vi "MB_TCP_7018_po.vi"(6 "N":i32, 9 "timeouts":T1={"conn_timeout"=1000, "reconn_timeout"=3000, "N attempt max"=3, "t_reset_TTL"=120000, "write_timeout"=10, "read_timeout"=500, "period"=100} {"t_reset_TTL" min=10 max=240000 step=1; "period" min=10 max=100000 step=1; "read_timeout" min=10 max=60000 step=1; "write_timeout" min=1 max=60000 step=1; "N attempt max" min=1 max=5 step=1; "reconn_timeout" min=10 max=240000 step=1; "conn_timeout" min=10 max=240000}, 10 "write enable":bool=TRUE, 11 "stop":bool) -> (0 "error out":errorcluster, 2 "errors":u32, 3 "Z3":u32)   [LabVIEW 2019]
uses:
  NI_modbus_upd/NI_modbus_upd.lvlib
  NI_modbus_upd.llb/MB Modbus Command.ctl
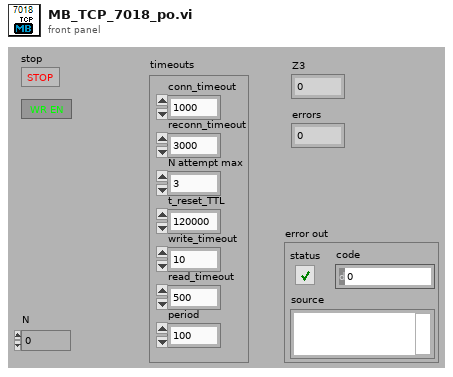
[diagram p1: front panel]
types:
  T1 = cluster{"conn_timeout":i32, "reconn_timeout":u32, "N attempt max":i32, "t_reset_TTL":u32, "write_timeout":i32, "read_timeout":i32, "period":u32}
  T2 = enum16{"Init", "Read", "Write", "Read inputs", "Read outputs"}
  T3 = enum16{"DI", "DO to write", "DO", "AI", "AO to write", "AO", "DI AI", "DI AO", "DO AI", "DO AO"}
  T4 = enum16{"Start", "Connect", "Write enable", "IP address", "Errors"}
  T5 = cluster{"Transaction ID":u16, "Protocol ID":u16, "Length":u16, "Unit ID":u8}
  T6 = typedef "MB Modbus Command.ctl" = cluster{"Function Code":u8, "Starting Address":u16, "Quantity":u16, "Data":u16[], "Discrete":bool[]}
  T7 = cluster{"Remote IP Address":string, "Remote Port":u16}
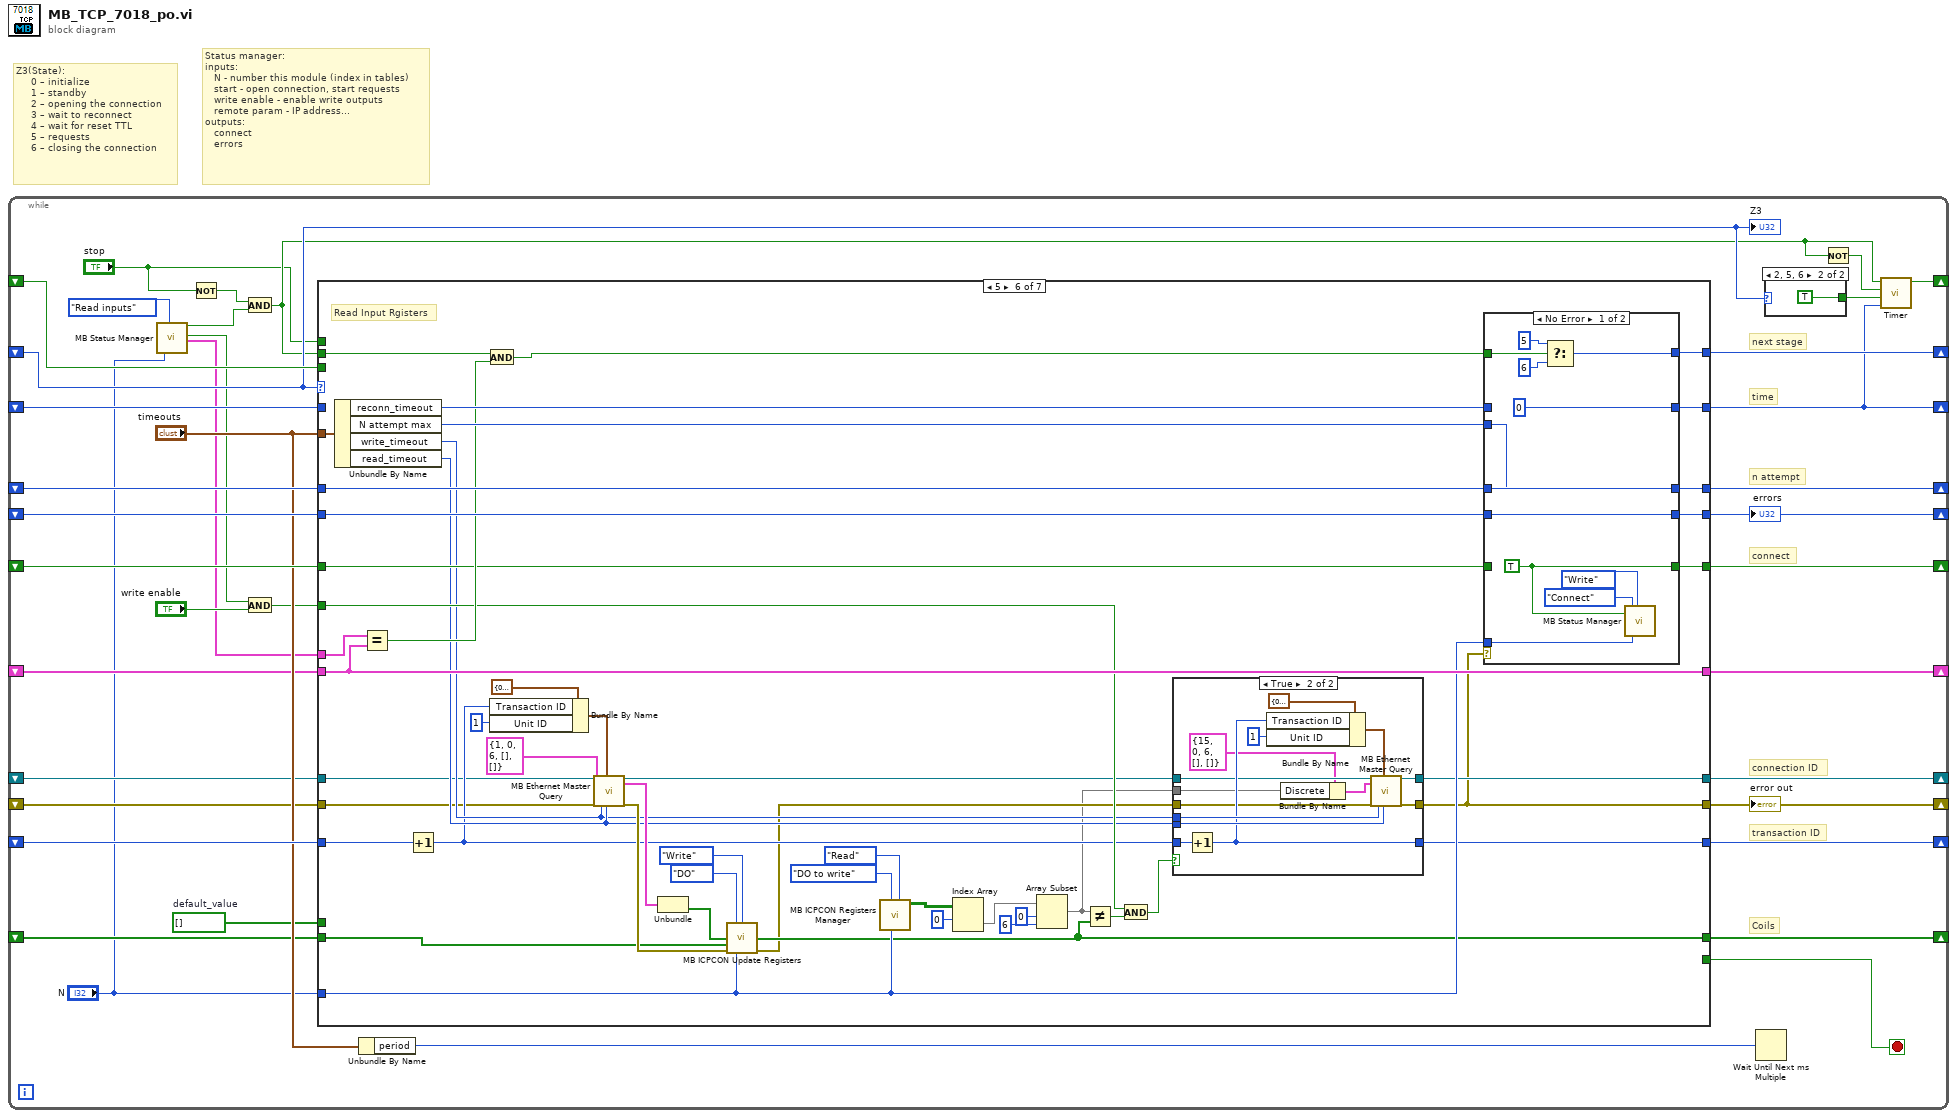
[diagram p0: block diagram]
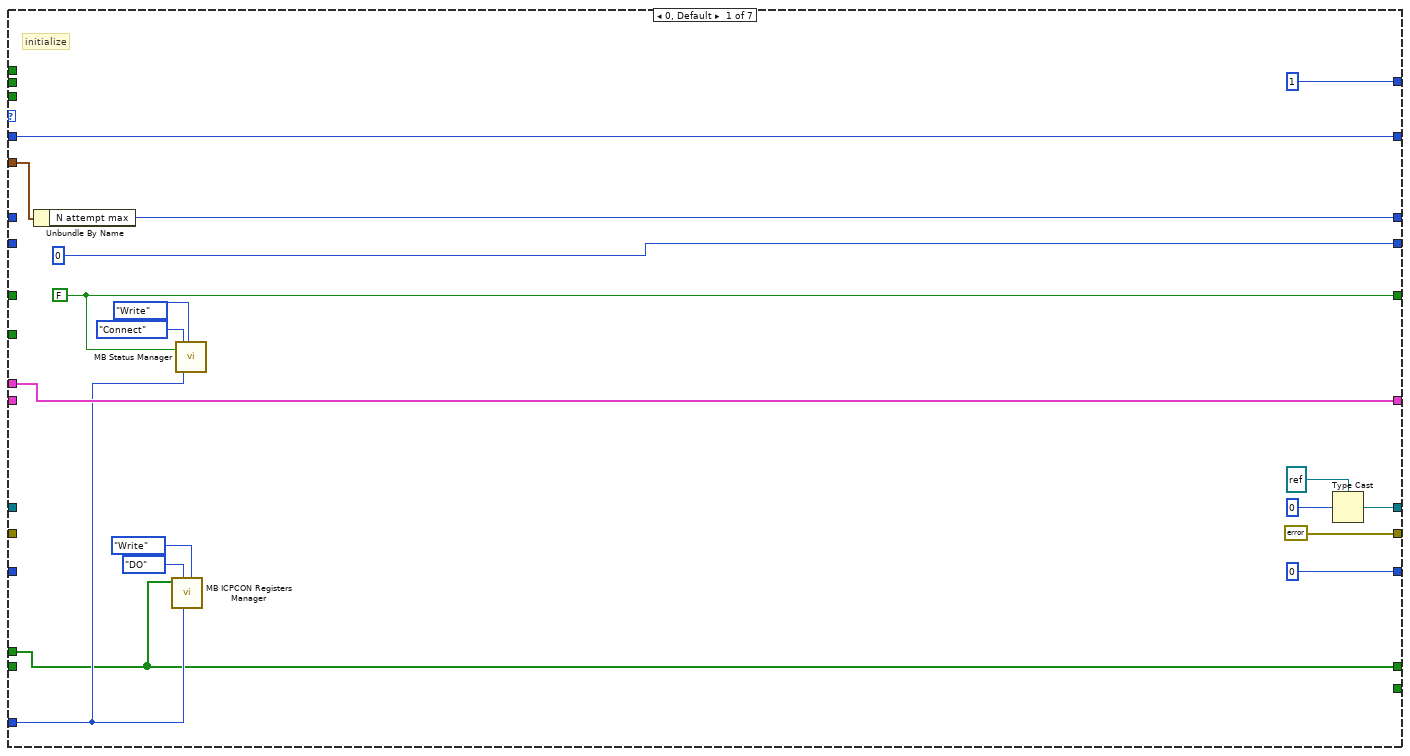
[diagram p2: hidden frame]
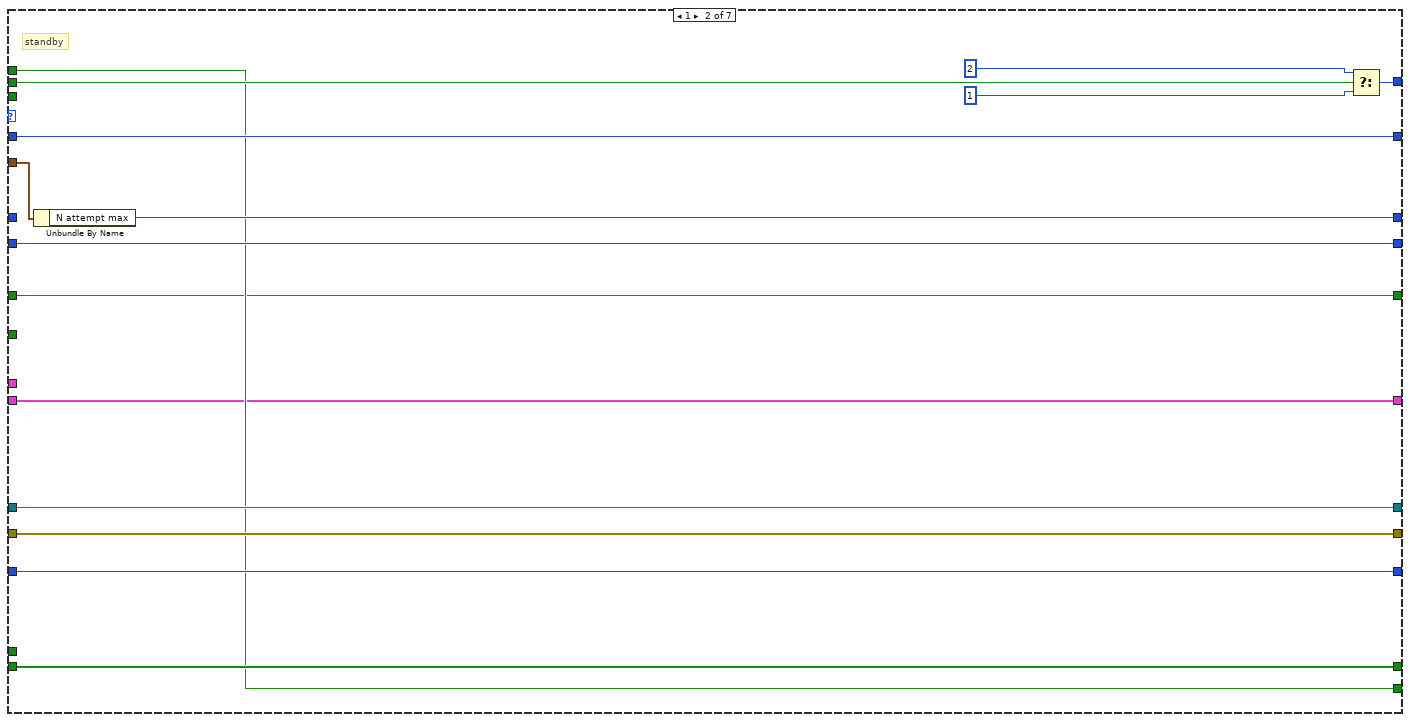
[diagram p3: hidden frame]
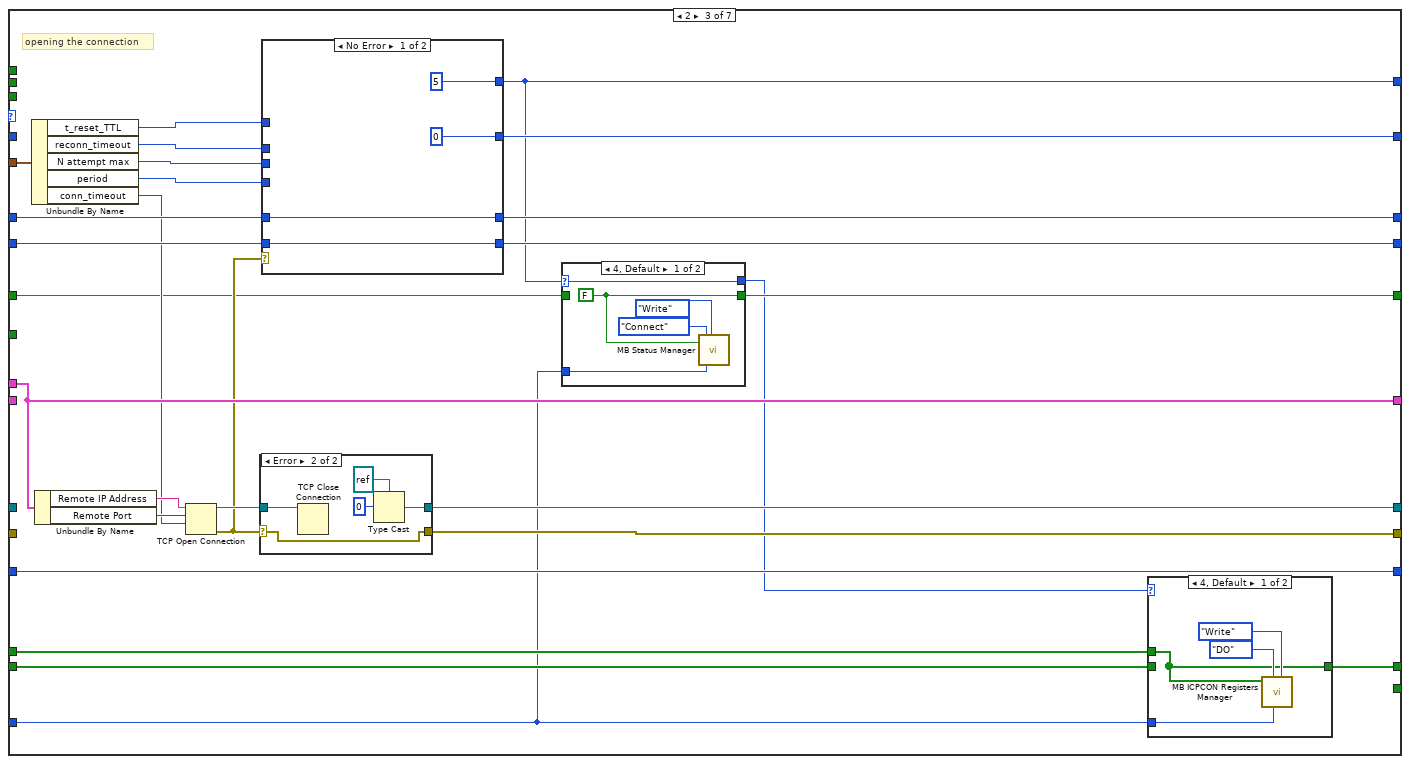
[diagram p4: hidden frame]
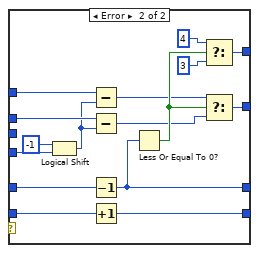
[diagram p7: hidden frame]
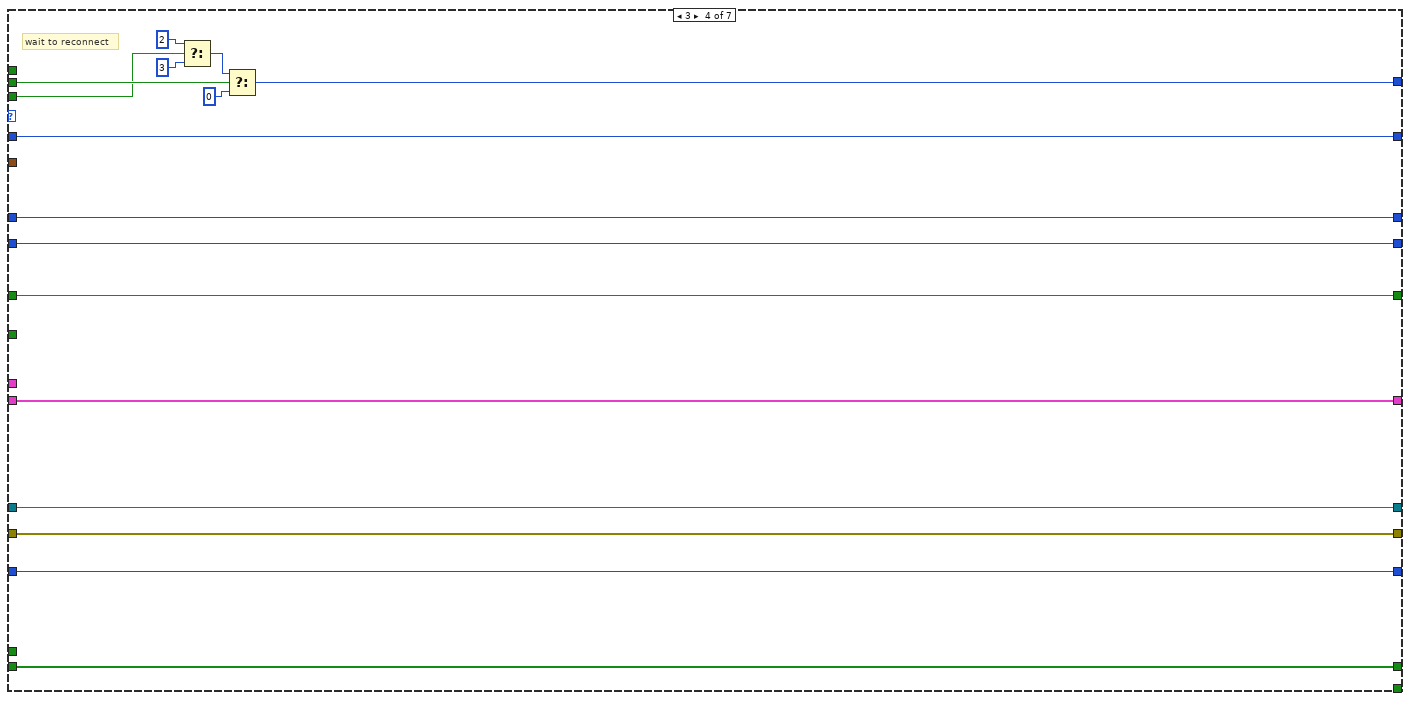
[diagram p9: hidden frame]
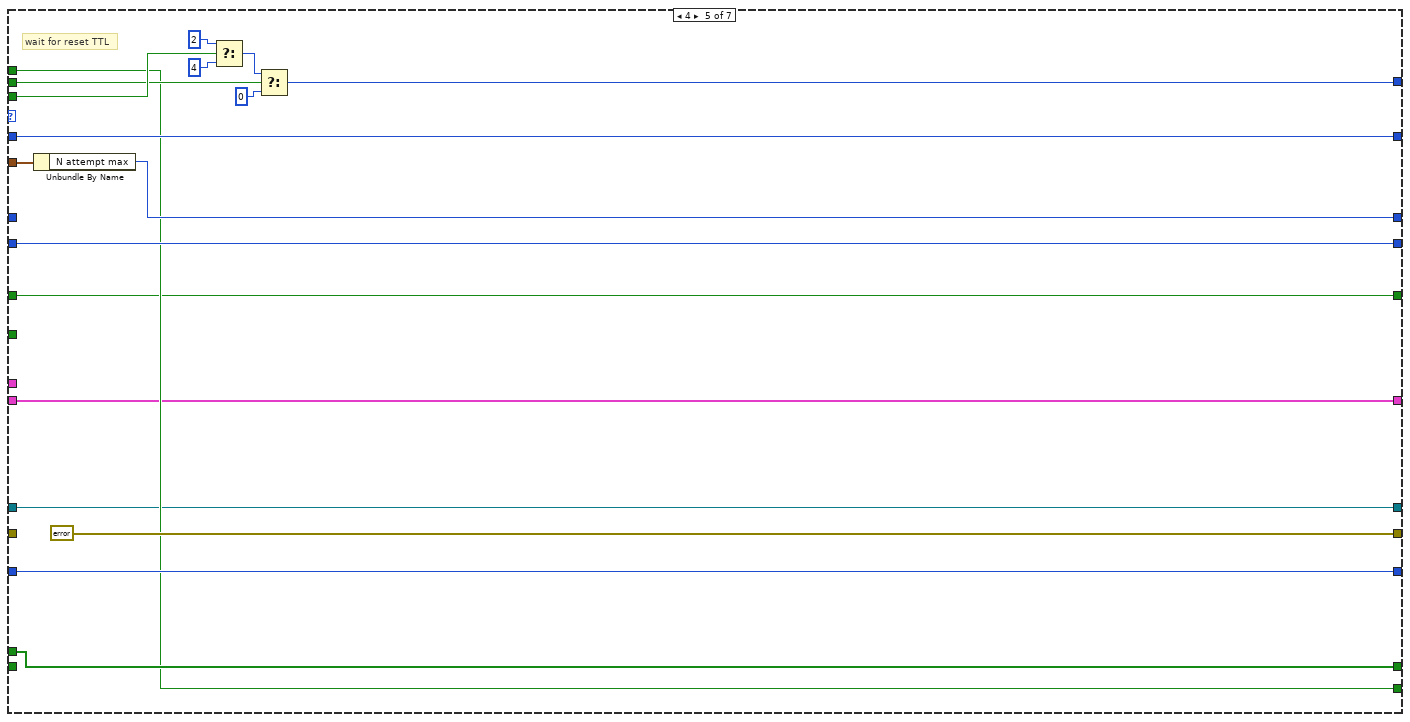
[diagram p10: hidden frame]
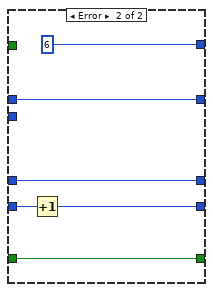
[diagram p12: hidden frame]
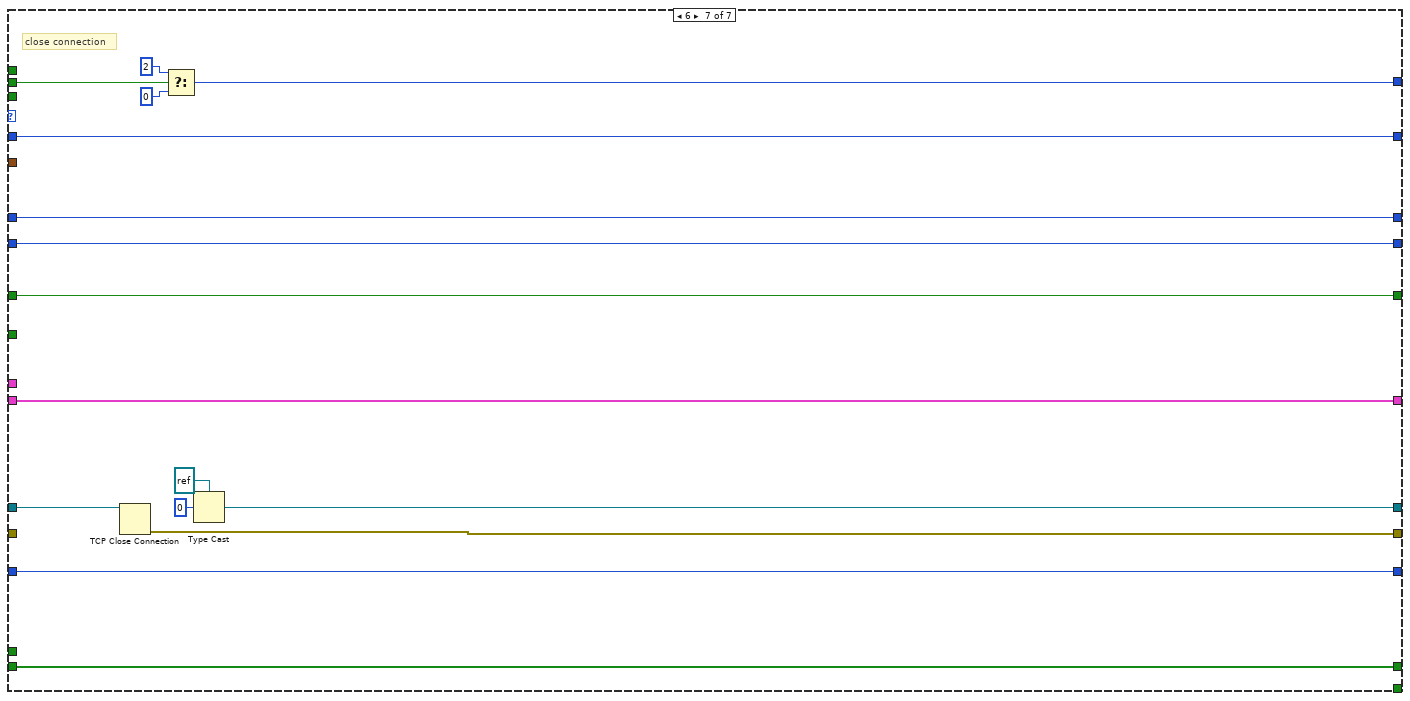
[diagram p13: hidden frame]
diagram:
  # "Status manager:\ninputs:\n   N - number this module (index in tables)\n   start - open connection, start requests\n   write enable - enable write outputs\n   remote param - IP address...\noutputs:\n   connect\n   errors"
  # "Z3(State):\n     0 – initialize \n     1 – standby\n     2 – opening the connection\n     3 – wait to reconnect\n     4 – wait for reset TTL\n     5 – requests\n     6 – closing the connection"
  n1 = while {
    shift-right: [w18] -> _
    shift-left: _ -> [w14]
    shift-right: [w17] -> _
    shift-left: _ -> [w37]
    shift-right: [w36] -> _
    shift-left: _ -> [w34]
    shift-right: [w35] -> _
    shift-left: _ -> [w33]
    shift-right: [w32] -> _
    shift-left: _ -> [w31]
    shift-right: [w30] -> _
    shift-left: _ -> [w19]
    shift-right: [w29] -> _
    shift-left: _ -> [w20]
    shift-right: [w28] -> _
    shift-left: _ -> [w27]
    shift-right: [w22] -> _
    shift-left: _ -> [w21]
    shift-right: [w16] -> _
    shift-left: _ -> [w15]
    shift-right: [w7] -> _
    shift-left: _ -> [w6]
    stop <- w10 stop-if-true
    w23 = bool[] []  # default_value
    # "Coils"
    # "connect"
    # "connection ID"
    # "transaction ID"
    # "n attempt"
    # "time"
    # "next stage"
    n2 = call "MB Status Manager.vi"("N"="N", "Function"=T2."Read inputs") -> ("start"=w4:bool, "write enable"=w3:bool, "Remote Param"=w2:T7)  [unwired: 12 in, 3 out]
    n3 = Not(x="stop") -> (.not. x?=w12:bool)
    n4 = And(x=w12, y=w4) -> (x .and. y?=w13:bool)
    n5 = And(x=w3, y="write enable") -> (x .and. y?=w9:bool)
    n6 = case shown="5" w14 {
      tunnel: [w54 w63 w79 w151 w156 w181 w268] -> w30
      tunnel: [errorcluster {"status"=FALSE, "code"=0, "source"=""} ("error out") w62 w77 w150 errorcluster {"status"=FALSE, "code"=0, "source"=""} ("error out") w180 w269] -> w29
      tunnel: w19 -> [_ w63 _ w151 w156 w173 w265]
      tunnel: w20 -> [_ w62 _ w150 _ w174 _]
      tunnel: [w42 w58 w75 w139 w155 w206 w256] -> w32
      tunnel: w31 -> [_ w58 w76 w139 w155 w207 w256]
      tunnel: w2 -> [w46 _ w82 _ _ w212 _]
      tunnel: w27 -> [_ w71 w98 w153 w171 w172 w270]
      tunnel: [u16 0 ("x") w71 w98 w153 w171 w183 w270] -> w28
      tunnel: [w48 w67 w93 w152 w167 w219 w262] -> w36
      tunnel: w34 -> [_ _ w94 w152 _ w219 w262]
      tunnel: [u32 0 ("N attempt max") w70 w96 w149 w170 w218 w267] -> w35
      tunnel: w33 -> [_ w70 w97 w149 w170 w217 w267]
      tunnel: [w50 w69 w90 w148 w169 w214 w266] -> w17
      tunnel: w37 -> [w50 w69 _ w148 w169 _ w266]
      tunnel: "timeouts" -> [w49 w68 w95 _ w168 w220 _]
      tunnel: w13 -> [_ w60 _ w144 w158 w211 w263]
      tunnel: [u32 1 w64 w73 w140 w162 w213 w257] -> w18
      tunnel: w15 -> [_ _ _ w142 w161 _ _]
      tunnel: w23 -> [w39 _ w83 _ w159 _ _]
      tunnel: [w39 w61 w84 w141 w159 w187 w260] -> w22
      tunnel: w21 -> [_ w61 w85 w141 _ w176 w260]
      tunnel: "N" -> [w41 _ w74 _ _ w191 _]
      tunnel: "stop" -> [_ w59 _ _ w157 _ _]
      tunnel: [_ w59 _ _ w157 _ _] -> w10
      tunnel: w9 -> [_ _ _ _ _ w194 _]
      tunnel: [w46 w57 w82 w138 w154 w209 w255] -> w7
      tunnel: w6 -> [_ w57 _ w138 w154 w209 w255]
      frame 0, Default {
        w42 = FALSE ("connect")
        # "initialize"
        n7 = Unbundle By Name(w49) -> ("N attempt max"=w48:i32)
        n8 = call "MB ICPCON Registers Manager.vi"("Function"=enum16{"Init", "Read", "Write", "Read All"}."Write", "N"=w41, "Table"=T3."DO", "Discrete in"=w39) -> ()  [unwired: 5 in, 3 out]
        n9 = call "MB Status Manager.vi"("connect in"=w42, "Table"=T4."Connect", "N"=w41, "Function"=T2."Write") -> ()  [unwired: 10 in, 6 out]
        n10 = Type Cast(type=refnum<k5> refnum ("connection ID"), x=u32 0) -> (*(type *) &x=w54:refnum<k5>)
      }
      frame 1 {
        # "standby"
        n11 = Unbundle By Name(w68) -> ("N attempt max"=w67:i32)
        n12 = Select(t=u32 2, s=w60, f=u32 1) -> (s? t:f=w64:u32)
      }
      frame 2 {
        # "opening the connection"
        n13 = Unbundle By Name(w95) -> ("t_reset_TTL"=w89:u32, "reconn_timeout"=w91:u32, "N attempt max"=w92:i32, "period"=w86:u32, "conn_timeout"=w81:i32)
        n14 = Unbundle By Name(w82) -> ("Remote IP Address"=w88:string, "Remote Port"=w87:u16)
        n15 = TCP Open Connection(address=w88, remote port or service name=w87, timeout ms (60000)=w81) -> (connection ID=w80:refnum<k5>, error out=w78:errorcluster)  [unwired: 2 in]
        n16 = case shown="Error" w78 {
          selector: w78 -> [w106 w108]
          tunnel: w80 -> [w107 w111]
          tunnel: [w107 w110] -> w79
          tunnel: [w106 w108] -> w77
          frame No Error {
          }
          frame Error {
            n17 = TCP Close Connection(connection ID=w111) -> ()  [unwired: 2 in, 2 out]
            n18 = Type Cast(type=refnum<k5> refnum ("connection ID"), x=u32 0) -> (*(type *) &x=w110:refnum<k5>)
          }
        }
        n19 = case shown="No Error" w78 {
          tunnel: w97 -> [w116 w132]
          tunnel: [w116 w131] -> w96
          tunnel: w94 -> [w115 w130]
          tunnel: [w115 w129] -> w93
          tunnel: w92 -> [_ _]
          tunnel: [u32 5 w126] -> w73
          tunnel: w91 -> [_ w125]
          tunnel: [u32 0 w124] -> w90
          tunnel: w89 -> [_ w121]
          tunnel: w86 -> [_ w119]
          frame No Error {
          }
          frame Error {
            n20 = Logical Shift(y=i16 -1, x=w119) -> (x << y=w117:u32)
            n21 = Subtract(x=w121, y=w117) -> (x-y=w120:u32)
            n22 = Subtract(x=w125, y=w117) -> (x-y=w122:u32)
            n23 = Decrement(x=w130) -> (x-1=w129:i32)
            n24 = Increment(x=w132) -> (x+1=w131:u32)
            n25 = Less Or Equal To 0?(x=w129) -> (x <= 0?=w123:bool)
            n26 = Select(t=u32 4, s=w123, f=u32 3) -> (s? t:f=w126:u32)
            n27 = Select(t=w120, s=w123, f=w122) -> (s? t:f=w124:u32)
          }
        }
        n28 = case shown="4, Default" w73 {
          selector: w73 -> [w99 w104]
          tunnel: w74 -> [w100 _]
          tunnel: [w101 w105] -> w75
          tunnel: w76 -> [_ w105]
          tunnel: [w99 w104] -> w72
          frame 4, Default {
            w101 = FALSE ("f")
            n29 = call "MB Status Manager.vi"("connect in"=w101, "Table"=T4."Connect", "N"=w100, "Function"=T2."Write") -> ()  [unwired: 10 in, 6 out]
          }
          frame 3, 5 {
          }
        }
        n30 = case shown="4, Default" w72 {
          tunnel: w74 -> [w135 _]
          tunnel: w85 -> [_ w137]
          tunnel: [w133 w137] -> w84
          tunnel: w83 -> [w133 _]
          frame 4, Default {
            n31 = call "MB ICPCON Registers Manager.vi"("Function"=enum16{"Init", "Read", "Write", "Read All"}."Write", "N"=w135, "Table"=T3."DO", "Discrete in"=w133) -> ()  [unwired: 5 in, 3 out]
          }
          frame 3, 5 {
          }
        }
      }
      frame 3 {
        # "wait to reconnect"
        n32 = Select(t=u32 2, s=w142, f=u32 3) -> (s? t:f=w143:u32)
        n33 = Select(t=w143, s=w144, f=u32 0) -> (s? t:f=w140:u32)
      }
      frame 4 {
        # "wait for reset TTL"
        n34 = Unbundle By Name(w168) -> ("N attempt max"=w167:i32)
        n35 = Select(t=u32 2, s=w161, f=u32 4) -> (s? t:f=w163:u32)
        n36 = Select(t=w163, s=w158, f=u32 0) -> (s? t:f=w162:u32)
      }
      frame 5 {
        # "Read Input Rgisters"
        n37 = Unbundle By Name(w220) -> ("reconn_timeout"=w215:u32, "N attempt max"=w216:i32, "write_timeout"=w185:i32, "read_timeout"=w186:i32)
        n38 = Equal?(x=w212, y=w209) -> (x = y?=w208:bool)
        n39 = Increment(x=w172) -> (x+1=w184:u16)
        n40 = And(x=w211, y=w208) -> (x .and. y?=w210:bool)
        n41 = Bundle By Name(cluster=T5 {"Transaction ID"=0, "Protocol ID"=0, "Length"=0, "Unit ID"=0} ("MBAP Header"), "Transaction ID"=w184, "Unit ID"=u8 1) -> (w203:T5)
        n42 = call "MB Ethernet Master Query.vi"("TCP Connection Refnum in"=w173, "Modbus Command"=T6 {"Function Code"=1, "Starting Address"=0, "Quantity"=6, "Data"=[], "Discrete"=[]} ("MODBUS Command"), "error in (no error)"=w174, "Write Timeout"=w185, "MBAP Header"=w203, "Read Timeout"=w186) -> ("TCP Connection Refnum (dup)"=w179:refnum<k5>, "Registers"=w198:cluster{"Registers":u16[], "Discrete":bool[]}, "error out"=w199:errorcluster)  [unwired: 9 in, 2 out]
        n43 = Unbundle(w198) -> ("Discrete"=w177:bool[])  [unwired: 1 out]
        n44 = call "MB ICPCON Update Registers.vi"("Table"=T3."DO", "Function"=enum16{"Init", "Read", "Write", "Read All"}."Write", "Discrete in"=w177, "Default Discrete in"=w176, "error in (no error)"=w199, "N"=w191) -> ("Discretes"=w187:bool[], "error out"=w178:errorcluster)  [unwired: 7 in, 1 out]
        n45 = call "MB ICPCON Registers Manager.vi"("Function"=enum16{"Init", "Read", "Write", "Read All"}."Read", "N"=w191, "Table"=T3."DO to write") -> ("Discretes"=w190:bool[][])  [unwired: 6 in, 2 out]
        n46 = Index Array(array=w190, index (row)=0) -> (element=w188:bool[])  [unwired: 1 in]
        n47 = Array Subset(array=w188, index=0, length=6) -> (w175:bool[])
        n48 = Not Equal?(x=w175, y=w187) -> (x != y?=w197:bool)
        n49 = And(x=w194, y=w197) -> (x .and. y?=w182:bool)
        n50 = case shown="True" w182 {
          tunnel: w186 -> [_ w235]
          tunnel: w185 -> [_ w234]
          tunnel: w184 -> [w222 w233]
          tunnel: [w222 w232] -> w183
          tunnel: w178 -> [w221 w230]
          tunnel: [w221 w229] -> w180
          tunnel: w179 -> [w223 w228]
          tunnel: [w223 w227] -> w181
          tunnel: w175 -> [_ w224]
          frame False {
          }
          frame True {
            n51 = Increment(x=w233) -> (x+1=w232:u16)
            n52 = Bundle By Name(cluster=T5 {"Transaction ID"=0, "Protocol ID"=0, "Length"=0, "Unit ID"=0} ("MBAP Header"), "Transaction ID"=w232, "Unit ID"=u8 1) -> (w236:T5)
            n53 = Bundle By Name(cluster=T6 {"Function Code"=15, "Starting Address"=0, "Quantity"=6, "Data"=[], "Discrete"=[]} ("MODBUS Command"), "Discrete"=w224) -> (w225:T6)
            n54 = call "MB Ethernet Master Query.vi"("TCP Connection Refnum in"=w228, "Modbus Command"=w225, "error in (no error)"=w230, "Write Timeout"=w234, "MBAP Header"=w236, "Read Timeout"=w235) -> ("TCP Connection Refnum (dup)"=w227:refnum<k5>, "error out"=w229:errorcluster)  [unwired: 9 in, 3 out]
          }
        }
        n55 = case shown="No Error" w180 {
          tunnel: w217 -> [w242 w254]
          tunnel: [w242 w253] -> w218
          tunnel: [w244 u32 6] -> w213
          tunnel: w219 -> [_ w251]
          tunnel: w216 -> [w248 _]
          tunnel: [w248 w251] -> _
          tunnel: w215 -> [_ w250]
          tunnel: [u32 0 w250] -> w214
          tunnel: w210 -> [w243 _]
          tunnel: w207 -> [_ w249]
          tunnel: [w239 w249] -> w206
          tunnel: w191 -> [w238 _]
          frame No Error {
            w239 = TRUE ("f")
            n56 = Select(t=u32 5, s=w243, f=u32 6) -> (s? t:f=w244:u32)
            n57 = call "MB Status Manager.vi"("connect in"=w239, "Table"=T4."Connect", "N"=w238, "Function"=T2."Write") -> ()  [unwired: 10 in, 6 out]
          }
          frame Error {
            n58 = Increment(x=w254) -> (x+1=w253:u32)
          }
        }
      }
      frame 6 {
        # "close connection"
        n59 = TCP Close Connection(connection ID=w265) -> (error out=w269:errorcluster)  [unwired: 2 in, 1 out]
        n60 = Select(t=u32 2, s=w263, f=u32 0) -> (s? t:f=w257:u32)
        n61 = Type Cast(type=refnum<k5> refnum ("connection ID"), x=u32 0) -> (*(type *) &x=w268:refnum<k5>)
      }
    }
    "error out" <- w29
    "errors" <- w35
    n62 = Unbundle By Name("timeouts") -> ("period"=w25:u32)
    n63 = Wait Until Next ms Multiple(millisecond multiple=w25) -> ()  [unwired: 1 out]
    n64 = case shown="2, 5, 6" w14 {
      tunnel: [_ TRUE] -> w24
      frame 0, Default {
      }
      frame 2, 5, 6 {
      }
    }
    n65 = Not(x=w13) -> (.not. x?=w38:bool)
    n66 = call "Timer.vi"("ms"=w17, "Load (F)"=w24, "Reset (F)"=w38, "Start (T)"=w13) -> ("End"=w16:bool)  [unwired: 5 in, 1 out]
    "Z3" <- w14
  }
